vi "get_variable_info.vi"(6 "timeout (25000ms)":i32=25000, 8 "error in (no error)":errorcluster, 9 "firmware information":string(combo)="variables", 11 "daemon reference in":refnum<k5>) -> (0 "error out":errorcluster, 1 "Size":i32, 2 "Address":i32, 3 "daemon reference out":refnum<k5>, 5 "command out":string="random")   [LabVIEW 2017]
doc: "<b>Command: </b>\"get_variable_info\"\n\n<b>Description: </b>This command extracts the variable information of the specified named variable.\n\n<b>Parameters: </b> \n\n 1. Variable Name\n\n<b>Note: </b>Make sure to use \"load_firmware_json\" command first to load the firmware file into the Daemon, otherwise this command will return no variable information.\n____________________________________________\nDIPC 692 Daemon API 10.0.0.1\nSam Tee - Dyson Technology Ltd\nCopyright (c) 2024, Dyson Technology Ltd"
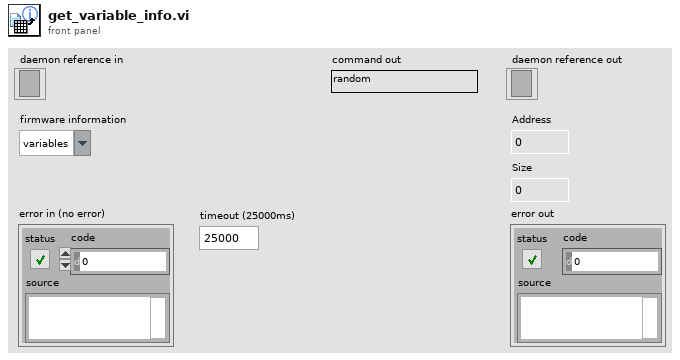
[diagram p1: front panel]
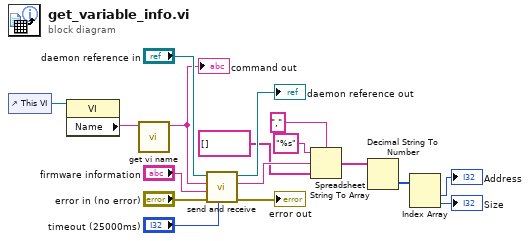
[diagram p0: block diagram]
diagram:
  n1 = control-ref of="This VI"() -> (w12:refnum<vi>)
  n2 = property class="VI"(reference=w12) -> ("Name"=w11:string)  [unwired: 1 in, 2 out]
  n3 = call "get vi name.vi"("library.lvlib:name.vi"=w11) -> ("vi name"=w10:string)  [unwired: 10 in]
  "command out" <- w10
  n4 = call "send and receive.vi"("timeout (25000ms)"="timeout (25000ms)", "error in (no error)"="error in (no error)", "data"="firmware information", "command"=w10, "daemon reference in"="daemon reference in") -> ("error out"=→"error out":errorcluster, "response"=w9:string, "daemon reference out"=→"daemon reference out":refnum<k5>)  [unwired: 4 in]
  n5 = Spreadsheet String To Array(delimiter (Tab)=",", format string="%s", spreadsheet string=w9, array type (2D Dbl)=string[] []) -> (array=w4:string[])
  n6 = Decimal String To Number(string=w4) -> (number=w3:i32[])  [unwired: 2 in, 1 out]
  n7 = Index Array(array=w3) -> (element #1=→"Address":i32, element #2=→"Size":i32)  [unwired: 2 in]
